vi "Main - Call and Monitor TCP Traffic.vi"() -> ()   [LabVIEW 2017, in "Multi-Loop Module Example.lvlib"]
uses:
  Multi-Loop Module Example.lvlib
  user.lib/_NEVSTOP/Communicable State Machine(CSM)/_Support/Common/Format Timestamp.vi
  user.lib/_NEVSTOP/Communicable State Machine(CSM)/Communicable State Machine.lvlib
panel:
  in  "String":string
  out "String Cache":string
  # "Overview:\n\nDemonstrates how to invoke the CSM submodule a side loop. Externally, this process is indistinguishable from other submodules based on CSM. What requires attention are the API and status changes.\n\nInstructions::\n\n1. Run this VI.\n2. Run the slightly modified Simple TCP - Client.vi, which is based on the LabVIEW example.\n3. Modify the String control on both this front panel and the client, and observe the log information.\n4. You can restart Simple TCP - Client.vi to view the logs."
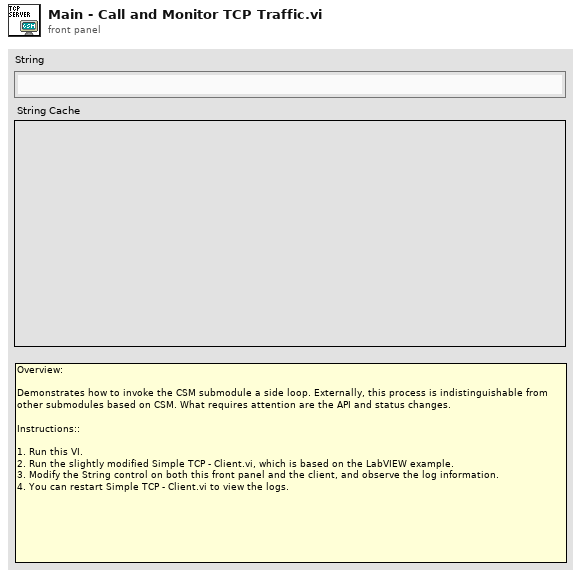
[diagram p1: front panel]
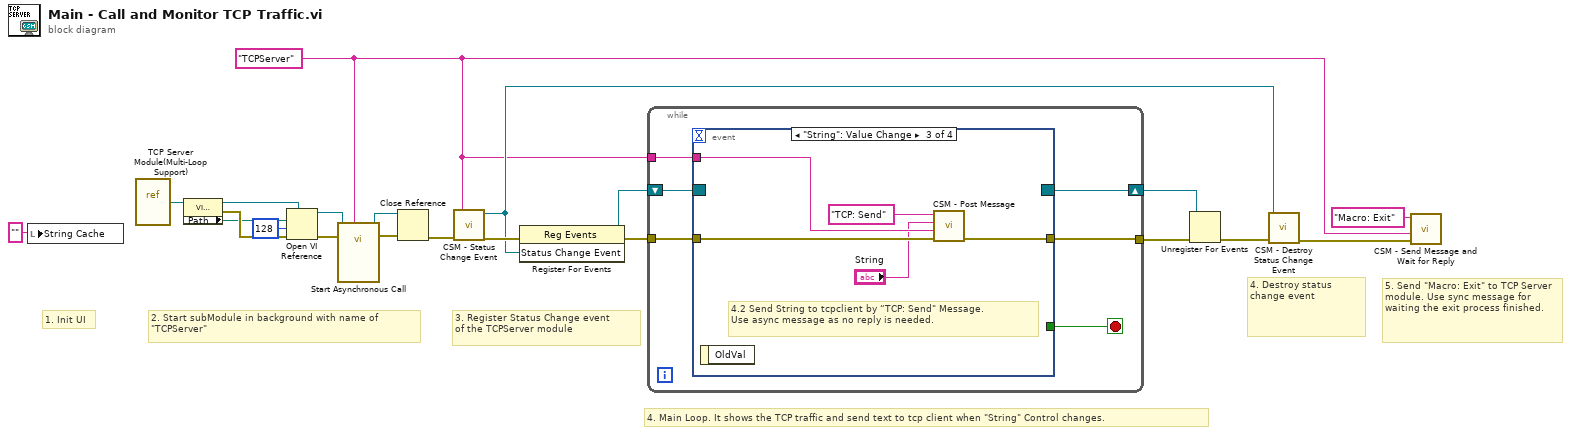
[diagram p0: block diagram]
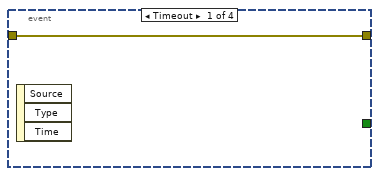
[diagram p2: hidden frame]
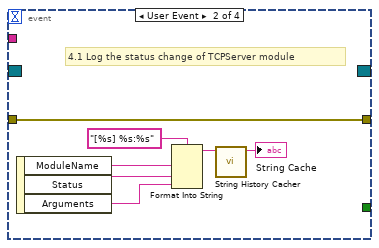
[diagram p3: hidden frame]
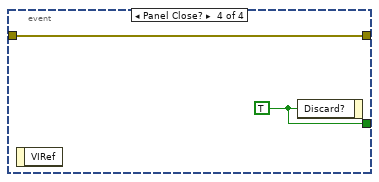
[diagram p4: hidden frame]
diagram:
  w6 = "TCPServer" ("Name (\"\" to Use UUID)")
  # "5. Send \"Macro: Exit\" to TCP Server module. Use sync message for waiting the exit process finished."
  # "4. Destroy status change event"
  # "4. Main Loop. It shows the TCP traffic and send text to tcp client when \"String\" Control changes."
  # "3. Register Status Change event\nof the TCPServer module"
  # "2. Start subModule in background with name of \"TCPServer\""
  # "1. Init UI"
  n1 = local write "String Cache"("" ("String Cache")) -> ()
  n2 = vi-ref "TCP Server Module(Multi-Loop Support).vi"() -> (w14:refnum<vi>)
  n3 = property class="VI (strict)"(reference=w14) -> (reference out=w18:refnum<vi>, error out=w16:errorcluster, "Path"=w15:path)  [unwired: 1 in]
  n4 = Open VI Reference(type specifier VI Refnum (for type only)=w18, vi path=w15, options=128, error in (no error)=w16) -> (vi reference=w17:refnum<vi>, error out=w13:errorcluster)  [unwired: 2 in]
  n5 = call-by-ref "Start Asynchronous Call"(reference=w17, error in=w13, "Name(\"\" to use uuid)"=w6) -> (reference out=w20:refnum<vi>, error out=w19:errorcluster)  [unwired: 11 in]
  n6 = Close Reference(reference=w20, error in (no error)=w19) -> (error out=w12:errorcluster)
  n7 = call "CSM - Status Change Event.vi"("Error In"=w12, "CSM Module"=w6) -> ("error out"=w11:errorcluster, "Status Change Event"=w8:refnum<user-event>)  [unwired: 7 in, 1 out]
  n8 = register-events(error in=w11, w8) -> (reference out=w9:refnum<event-registration>, error out=w10:errorcluster)  [unwired: 1 in]
  n9 = while {
    tunnel: w10 -> [w24]
    tunnel: [w25] -> w3
    tunnel: w6 -> [w23]
    shift-right: [w22] -> w1
    shift-left: w9 -> [w26]
    stop <- w27 stop-if-true
    n10 = event shown="[2] \"String\": Value Change" {
      selector: w26 -> [_ _ _ _]
      dyn-events: [_ _ _ _] -> w22
      timeout: _ -> [_ _ _ _]
      tunnel: [_ _ _ w42] -> w27
      tunnel: [w28 w35 w39 w41] -> w25
      tunnel: w24 -> [w28 w35 w40 w41]
      tunnel: w23 -> [_ _ w38 _]
      event Timeout {
        n11 = event-data() -> ()  [unwired: 1 in, 3 out]
      }
      event User Event {
        # "4.1 Log the status change of TCPServer module"
        n12 = event-data() -> ("ModuleName"=w34:string, "Status"=w33:string, "Arguments"=w32:string)  [unwired: 1 in]
        n13 = Format Into String(format string="[%s] %s:%s", w34, w33, w32) -> (resulting string=w30:string)  [unwired: 2 in, 1 out]
        n14 = call "String History Cacher.vi"("String"=w30) -> ("String Cache"=→"String Cache":string)  [unwired: 10 in]
      }
      event "String": Value Change {
        # "4.2 Send String to tcpclient by “TCP: Send\" Message.\nUse async message as no reply is needed."
        n15 = event-data() -> ()  [unwired: 1 in, 1 out]
        n16 = call "CSM - Post Message.vi"("Error In (No Error)"=w40, "Target Module"=w38, "Arguments (\"\")"="String", "State"="TCP: Send") -> ("error out"=w39:errorcluster)  [unwired: 7 in]
      }
      event Panel Close? {
        w42 = TRUE ("Discard?")
        n17 = event-data() -> ()  [unwired: 1 in, 1 out]
        n18 = event-data("Discard?"=w42) -> ()  [unwired: 1 in, 1 out]
      }
    }
  }
  n19 = Unregister For Events(event registration refnum=w1, error in=w3) -> (error out=w2:errorcluster)
  n20 = call "CSM - Destroy Status Change Event.vi"("Error In"=w2, "Status Change Event"=w8) -> ("error out"=w7:errorcluster)  [unwired: 9 in]
  n21 = call "CSM - Send Message and Wait for Reply.vi"("Error In (No Error)"=w7, "Target Module"=w6, "State"="Macro: Exit") -> ()  [unwired: 6 in, 3 out]
